vi "Pound.vi"(9 "number of rotations":dbl, 10 "item to pound":refnum<class "Poundable.lvclass">, 11 "Pounding Tool in":refnum<class "Pounding Tool.lvclass">) -> (2 "pounded item":refnum<class "Poundable.lvclass">)   [LabVIEW 2023, in "Pounding Tool.lvclass"]
uses:
  Pounding Tool.lvclass
  Poundable/Poundable.lvclass
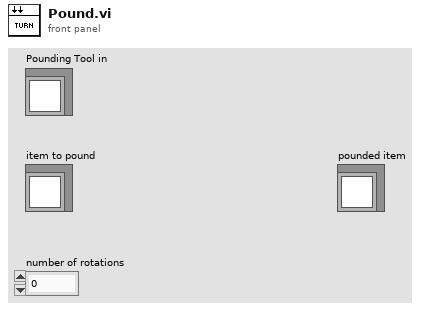
[diagram p1: front panel]
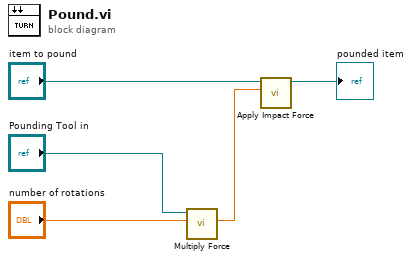
[diagram p0: block diagram]
diagram:
  n1 = call-dynamic "Multiply Force.vi"("force in"="number of rotations", "Pounding Tool"="Pounding Tool in") -> ("force out"=w1:dbl)  [unwired: 9 in]
  n2 = call-dynamic "Apply Impact Force.vi"("force"=w1, "Poundable in"="item to pound") -> ("Poundable out"=→"pounded item":refnum<class "Poundable.lvclass">)  [unwired: 9 in]
